vi "Keithley2400series_Close.vi"(0 "error in (no error)":errorcluster, 1 "VISA resource name":refnum<visa-resource-name>) -> ()   [LabVIEW 2014]
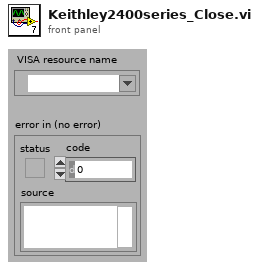
[diagram p1: front panel]
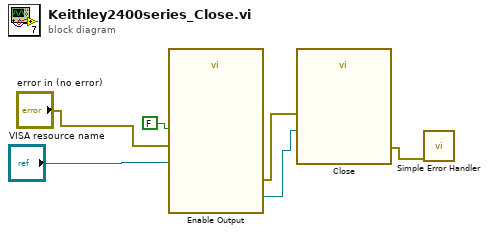
[diagram p0: block diagram]
diagram:
  n1 = call "Enable Output.vi"("error in (no error)"="error in (no error)", "Enable Output (T: Enable)"=FALSE, "VISA resource name"="VISA resource name") -> ("error out"=w2:errorcluster, "VISA resource name out"=w3:refnum<visa-resource-name>)  [unwired: 7 in]
  n2 = call "Close.vi"("error in (no error)"=w2, "VISA resource name"=w3) -> ("error out"=w4:errorcluster)  [unwired: 9 in]
  n3 = call <vilib>:"Simple Error Handler.vi"("error in (no error)"=w4) -> ()  [unwired: 4 in, 5 out]
